vi "Unpack TCP Message.vi"(11 "data in":string) -> (0 "LabVIEW Server ID":string, 1 "Script ID":i64, 2 "Data":string, 3 "Command":string, 4 "Python Message ID":i32)   [LabVIEW 2013, in "TS.lvlib"]
doc: "This VI assumes the input looks like this:\nCommand|[\"first data\",\"second data\"]\nand pushes the \"command\" string into the first output, and the list or array into the Data output."
uses:
  TS.lvlib
panel:
  # "This VI assumes the input looks like this:\nCommand|[\"first data\",\"second data\"]\nand pushes the \"command\" string into the first output, and the list or array into the Data output."
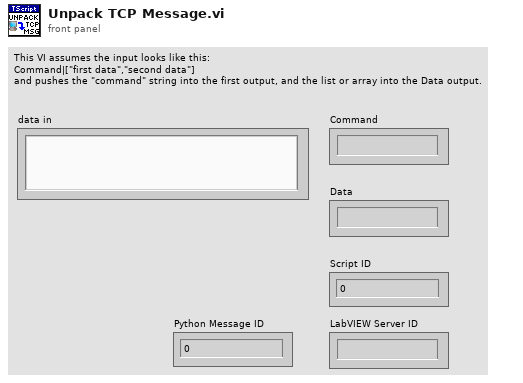
[diagram p1: front panel]
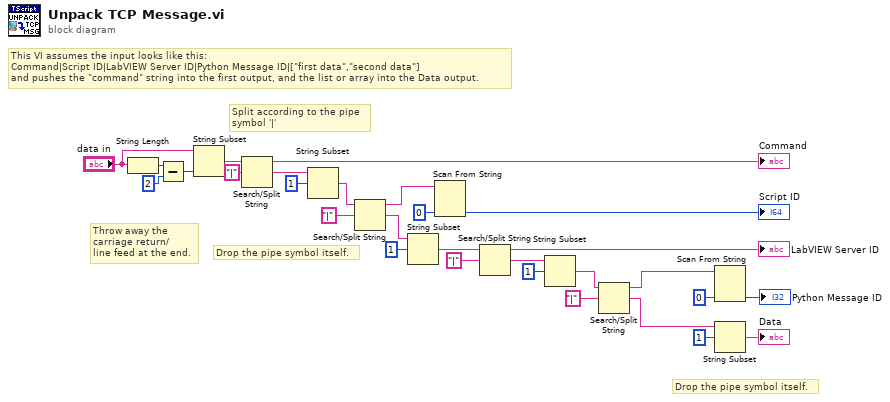
[diagram p0: block diagram]
diagram:
  # "Drop the pipe symbol itself."
  # "This VI assumes the input looks like this:\nCommand|Script ID|LabVIEW Server ID|Python Message ID|[\"first data\",\"second data\"]\nand pushes the \"command\" string into the first output, and the list or array into the Data output."
  # "Drop the pipe symbol itself."
  # "Split according to the pipe\nsymbol '|'"
  # "Throw away the\ncarriage return/\nline feed at the end."
  n1 = String Length(string="data in") -> (length=w29:i32)
  n2 = Subtract(x=w29, y=2) -> (x-y=w26:i32)
  n3 = String Subset(string="data in", length (rest)=w26) -> (substring=w25:string)  [unwired: 1 in]
  n4 = Search/Split String(string=w25, search string/char (-)="|") -> (substring before match=→"Command":string, match + rest of string=w15:string)  [unwired: 1 in, 1 out]
  n5 = String Subset(string=w15, offset (0)=1) -> (substring=w14:string)  [unwired: 1 in]
  n6 = Search/Split String(string=w14, search string/char (-)="|") -> (substring before match=w18:string, match + rest of string=w11:string)  [unwired: 1 in, 1 out]
  n7 = String Subset(string=w11, offset (0)=1) -> (substring=w10:string)  [unwired: 1 in]
  n8 = Scan From String(input string=w18, default 1=i64 0) -> (output 1=→"Script ID":i64)  [unwired: 3 in, 3 out]
  n9 = Search/Split String(string=w10, search string/char (-)="|") -> (substring before match=→"LabVIEW Server ID":string, match + rest of string=w7:string)  [unwired: 1 in, 1 out]
  n10 = String Subset(string=w7, offset (0)=1) -> (substring=w3:string)  [unwired: 1 in]
  n11 = Search/Split String(string=w3, search string/char (-)="|") -> (substring before match=w2:string, match + rest of string=w1:string)  [unwired: 1 in, 1 out]
  n12 = Scan From String(input string=w2, default 1=0) -> (output 1=→"Python Message ID":i32)  [unwired: 3 in, 3 out]
  n13 = String Subset(string=w1, offset (0)=1) -> (substring=→"Data":string)  [unwired: 1 in]
